vi "Init Talon Drive Motors With CVS Files.vi"(2 "error in":errorcluster, 3 "Robot ID":string="985") -> (0 "error out":errorcluster, 1 "RobotDriveDevRef":T1)   [LabVIEW 2017]
uses:
  <vilib>/Rock Robotics/WPI/RobotDrive/WPI_RobotDriveDevRef.ctl
  <vilib>/Rock Robotics/WPI/MotorControl/WPI_MotorControlDeviceRef.ctl
  <vilib>/Rock Robotics/WPI/MotorControl/WPI_MotorControlType.ctl
  <vilib>/Rock Robotics/SystemInterfaces/DIO/FPGA_DIOPWMChannel.ctl
  <vilib>/Rock Robotics/WPI/PWM/WPI_PWMDeadband.ctl
  <vilib>/Rock Robotics/SystemInterfaces/DIO/FPGA_DIOChannel.ctl
  <vilib>/Rock Robotics/WPI/SafetyOutput/WPI_SafetyOutputConfigMenu.ctl
  <vilib>/Rock Robotics/WPI/RobotDrive/WPI_RobotDriveOpen4MotorWithExistingMotors.vi
  <vilib>/Rock Robotics/WPI/RobotDrive/WPI_RobotDriveOpen2MotorWithTalon.vi
panel:
  out "Drive Right Front":u8
  out "Drive Left Front":u8
  out "Drive Right Rear":u8
  out "Drive Left Rear":u8
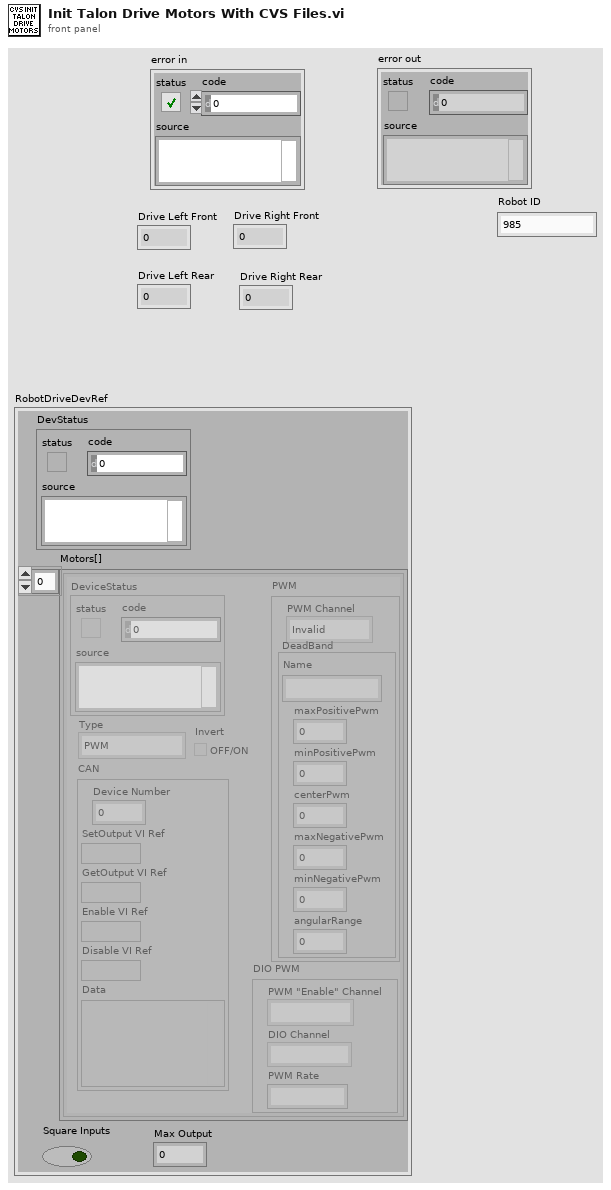
[diagram p1: front panel]
types:
  T1 = typedef "WPI_RobotDriveDevRef.ctl" = cluster{"DevStatus":errorcluster, "Motors[]":T2[], "Square Inputs":bool, "Max Output":dbl}
  T2 = typedef "WPI_MotorControlDeviceRef.ctl" = cluster{"DeviceStatus":errorcluster, "Type":T3, "PWM":cluster{"PWM Channel":T4, "DeadBand":T5}, "CAN":cluster{"Device Number":u8, "SetOutput VI Ref":variant, "GetOutput VI Ref":variant, "Enable VI Ref":variant, "Disable VI Ref":variant, "Data":variant}, "Invert":bool, "DIO PWM":cluster{"PWM \"Enable\" Channel":T4, "DIOChannel":T6, "PWM Rate":dbl}}
  T3 = typedef "WPI_MotorControlType.ctl" = enum16{"PWM", "CAN", "DIO PWM"}
  T4 = typedef "FPGA_DIOPWMChannel.ctl" = enum8{"PWM 0", "PWM 1", "PWM 2", "PWM 3", "PWM 4", "PWM 5", "PWM 6", "PWM 7", "PWM 8", "PWM 9", "PWM MXP 0", "PWM MXP 1", "PWM MXP 2", "PWM MXP 3", "PWM MXP 4", "PWM MXP 5", "PWM MXP 6", "PWM MXP 7", "PWM MXP 8", "PWM MXP 9", "Invalid"}
  T5 = typedef "WPI_PWMDeadband.ctl" = cluster{"Name":string, "maxPositivePwm":i32, "minPositivePwm":i32, "centerPwm":i32, "maxNegativePwm":i32, "minNegativePwm":i32, "angularRange":u16}
  T6 = typedef "FPGA_DIOChannel.ctl" = enum8{"DIO 0", "DIO 1", "DIO 2", "DIO 3", "DIO 4", "DIO 5", "DIO 6", "DIO 7", "DIO 8", "DIO 9", "DIO MXP 0", "DIO MXP 1", "DIO MXP 2", "DIO MXP 3", "DIO MXP 4", "DIO MXP 5", "DIO MXP 6", "DIO MXP 7", "DIO MXP 8", "DIO MXP 9", "DIO MXP 10", "DIO MXP 11", "DIO MXP 12", "DIO MXP 13", "DIO MXP 14", "DIO MXP 15", "SPI Port CS1", "SPI Port CS2", "SPI Port CS3", "SPI Port MISO", "SPI Port MOSI", "Invalid"}
  T7 = typedef "WPI_SafetyOutputConfigMenu.ctl" = enum16{"Enable", "Disable"}
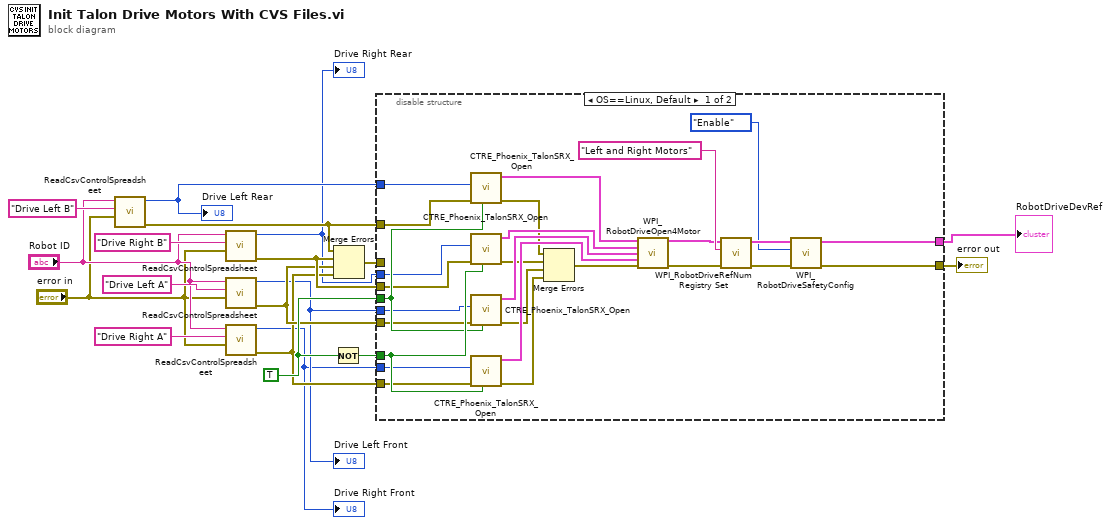
[diagram p0: block diagram]
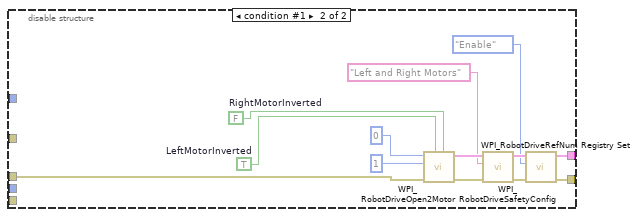
[diagram p2: hidden frame]
diagram:
  w14 = TRUE ("Invert")
  n1 = call "ReadCsvControlSpreadsheet.vi"("error in"="error in", "Motor ID"="Drive Left B", "Robot ID"="Robot ID") -> ("error out"=w9:errorcluster, "Can Bus ID"=w4:u8)  [unwired: 7 out]
  "Drive Left Rear" <- w4
  n2 = call "ReadCsvControlSpreadsheet.vi"("error in"="error in", "Motor ID"="Drive Right B", "Robot ID"="Robot ID") -> ("error out"=w8:errorcluster, "Can Bus ID"=w3:u8)  [unwired: 7 out]
  "Drive Right Rear" <- w3
  n3 = call "ReadCsvControlSpreadsheet.vi"("error in"="error in", "Motor ID"="Drive Left A", "Robot ID"="Robot ID") -> ("error out"=w7:errorcluster, "Can Bus ID"=w2:u8)  [unwired: 7 out]
  "Drive Left Front" <- w2
  n4 = call "ReadCsvControlSpreadsheet.vi"("error in"="error in", "Motor ID"="Drive Right A", "Robot ID"="Robot ID") -> ("error out"=w6:errorcluster, "Can Bus ID"=w1:u8)  [unwired: 7 out]
  "Drive Right Front" <- w1
  n5 = Not(x=w14) -> (.not. x?=w15:bool)
  n6 = Merge Errors(w9, w8, w7, w6) -> (w11:errorcluster)
  n7 = disable-structure shown="OS==Linux, Default" {
    disable-tunnel: w15 -> [w46 _]
    disable-tunnel: w14 -> [w45 _]
    disable-tunnel: w4 -> [w40 _]
    disable-tunnel: w3 -> [w39 _]
    disable-tunnel: w2 -> [w38 _]
    disable-tunnel: w1 -> [w37 _]
    disable-tunnel: [w31 w50] -> w12
    disable-tunnel: w11 -> [_ w49]
    disable-tunnel: [w20 w47] -> w10
    disable-tunnel: w9 -> [w30 _]
    disable-tunnel: w8 -> [w29 _]
    disable-tunnel: w7 -> [w28 _]
    disable-tunnel: w6 -> [w27 _]
    frame condition #0 (active) {
      n8 = call "CTRE_Phoenix_TalonSRX_Open.vi"("Invert"=w45, "error in"=w30, "Device Number"=w40) -> ("error out"=w26:errorcluster, "CAN Talon SRX Ref"=w41:T2)  [unwired: 7 in]
      n9 = call "CTRE_Phoenix_TalonSRX_Open.vi"("Invert"=w46, "error in"=w29, "Device Number"=w39) -> ("error out"=w25:errorcluster, "CAN Talon SRX Ref"=w42:T2)  [unwired: 7 in]
      n10 = call "CTRE_Phoenix_TalonSRX_Open.vi"("Invert"=w45, "error in"=w28, "Device Number"=w38) -> ("error out"=w24:errorcluster, "CAN Talon SRX Ref"=w43:T2)  [unwired: 7 in]
      n11 = call "CTRE_Phoenix_TalonSRX_Open.vi"("Invert"=w46, "error in"=w27, "Device Number"=w37) -> ("error out"=w23:errorcluster, "CAN Talon SRX Ref"=w44:T2)  [unwired: 7 in]
      n12 = Merge Errors(w26, w25, w24, w23) -> (w22:errorcluster)
      n13 = call-poly <vilib>:"WPI_RobotDriveOpen4Motor.vi"("Rear Left Motor Dev Ref"=w41, "Rear Right Motor Dev Ref"=w42, "Front Left Motor Dev Ref"=w43, "Front Right Motor Dev Ref"=w44, "error in (no error)"=w22) -> ("RobotDriveDevRef"=w33:T1, "error out"=w32:errorcluster)  [unwired: 9 in]
      n14 = call <vilib>:"WPI_RobotDriveRefNum Registry Set.vi"("error in (no error)"=w32, "refnum name"="Left and Right Motors", "RobotDriveDevRef"=w33) -> ("error out"=w21:errorcluster, "RobotDriveDevRef"=w36:T1)  [unwired: 1 in, 6 out]
      n15 = call <vilib>:"WPI_RobotDriveSafetyConfig.vi"("error in (no error)"=w21, "mode"=WPI_SafetyOutputConfigMenu."Enable", "RobotDriveDevRef"=w36) -> ("error out"=w20:errorcluster, "RobotDriveDevRef"=w31:T1)  [unwired: 7 in]
    }
    frame condition #1 {
      w54 = TRUE  # LeftMotorInverted
      w55 = FALSE  # RightMotorInverted
      n16 = call-poly <vilib>:"WPI_RobotDriveOpen2Motor.vi"("Right Motor Inverted"=w55, "Left Motor Inverted"=w54, "error in (no error)"=w49, "Right Motor"=u8 1 ("Left Motor"), "Left Motor"=u8 0) -> ("error out"=w58:errorcluster, "RobotDriveDevRef"=w57:T1)  [unwired: 5 out]
      n17 = call <vilib>:"WPI_RobotDriveRefNum Registry Set.vi"("error in (no error)"=w58, "refnum name"="Left and Right Motors", "RobotDriveDevRef"=w57) -> ("error out"=w48:errorcluster, "RobotDriveDevRef"=w59:T1)  [unwired: 1 in, 6 out]
      n18 = call <vilib>:"WPI_RobotDriveSafetyConfig.vi"("error in (no error)"=w48, "mode"=WPI_SafetyOutputConfigMenu."Enable", "RobotDriveDevRef"=w59) -> ("error out"=w47:errorcluster, "RobotDriveDevRef"=w50:T1)  [unwired: 7 in]
    }
  }
  "RobotDriveDevRef" <- w12
  "error out" <- w10
